vi "Item_OnPopupMenu.vi"(11 "Object":T1) -> ()   [LabVIEW 2020, in "Actor Message Maker Provider.lvlib"]
uses:
  Actor Message Maker Provider.lvlib
  <resource>/Framework/Providers/API/mxLvMenuItem.ctl
  MessageMakerProvider/Support/Localized Strings.vi
  MessageMakerProvider/Message Maker Provider.lvlib
  MessageMakerProvider/AFPP Shared/Validation Mode.ctl
  MessageMakerProvider/AFPP Shared/AFPP Shared.lvlib
  <resource>/Framework/Providers/API/ItemRef.ctl
panel:
  out "error out":errorcluster
  in  "error in":errorcluster
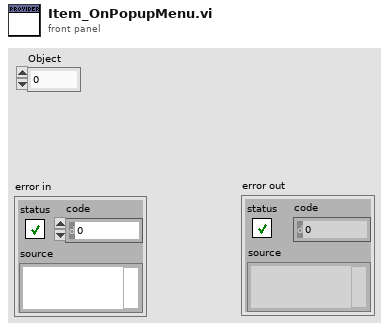
[diagram p1: front panel]
types:
  T1 = typedef "ItemRef.ctl" = u64
  T2 = typedef "AFPP Shared.lvlib/Validation Mode.ctl" = enum16{"An Actor Library", "A Target Tag"}
  T3 = typedef "mxLvMenuItem.ctl" = cluster{"Menu Name":string, "Description":string, "Icon File Name":path, "Menu Tag":string, "Enabled":bool, "Checked":bool, "Separator":bool, "Batchable":bool, "Weight":i32, "Batch Mode (Ignored if Not Batchable)":enum32{"Show If All Items Support Command", "Show If Any Items Support Command"}, "Menu Location":enum32{"<None>", "Project", "Project / Build Specifications", "Tools", "Tools / Source Control", "Tools / Real-Time Module", "Help"}, "Exclude From Getting Started Window Menu":bool}
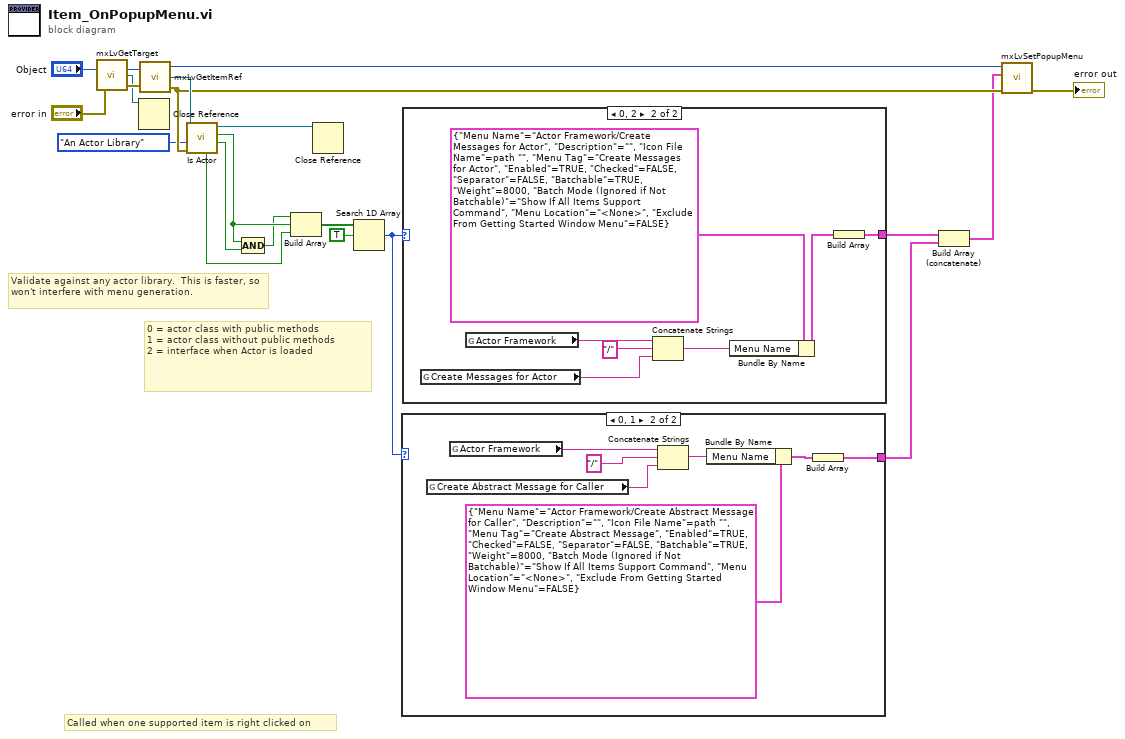
[diagram p0: block diagram]
diagram:
  # "0 = actor class with public methods\n1 = actor class without public methods\n2 = interface when Actor is loaded"
  # "Validate against any actor library.  This is faster, so won't interfere with menu generation."
  # "Called when one supported item is right clicked on"
  n1 = call <resource>:"mxLvGetTarget.vi"("Item"="Object", "error in"="error in") -> ("Item"=w10:T1, "Target"=w7:refnum<vi>, "error out"=w8:errorcluster)
  n2 = Close Reference(reference=w7) -> ()  [unwired: 1 in, 1 out]
  n3 = call <resource>:"mxLvGetItemRef.vi"("Item"=w10, "error in"=w8) -> ("Item"=w20:T1, "Item Refnum"=w18:refnum<vi>, "error out"=w17:errorcluster)
  n4 = call "Is Actor.vi"("error in (no error)"=w17, "Validation"=Validation_Mode."An Actor Library", "ProjectItem in"=w18) -> ("Has Public Methods"=w12:bool, "Is Actor"=w16:bool, "ProjectItem out"=w19:refnum<vi>, "Is Actor Interface"=w5:bool)  [unwired: 4 in, 1 out]
  n5 = Compound Arithmetic op=AND(w16, w12) -> (w15:bool)
  n6 = Build Array(w15, w16, w5) -> (w14:bool[])
  n7 = Close Reference(reference=w19) -> ()  [unwired: 1 in, 1 out]
  n8 = Search 1D Array(1D array=w14, element=TRUE) -> (index of element=w4:i32)  [unwired: 1 in]
  n9 = case shown="0, 1" w4 {
    tunnel: [_ w22] -> w2
    frame Default {
    }
    frame 0, 1 {
      n10 = global read "Localized Strings.vi" "Create Abstract Message for Caller"() -> (w26:string)
      n11 = global read "Localized Strings.vi" "Actor Framework"() -> (w25:string)
      n12 = Concatenate Strings(w25, "/", w26) -> (w27:string)
      n13 = Bundle By Name(cluster=T3 {"Menu Name"="Actor Framework/Create Abstract Message for Caller", "Description"="", "Icon File Name"=path "", "Menu Tag"="Create Abstract Message", "Enabled"=TRUE, "Checked"=FALSE, "Separator"=FALSE, "Batchable"=TRUE, "Weight"=8000, "Batch Mode (Ignored if Not Batchable)"=enum."Show If All Items Support Command", "Menu Location"=enum."<None>", "Exclude From Getting Started Window Menu"=FALSE} ("Menu Item"), "Menu Name"=w27) -> (w23:T3)
      n14 = Build Array(w23) -> (w22:T3[])
    }
  }
  n15 = case shown="0, 2" w4 {
    tunnel: [_ w33] -> w3
    frame Default {
    }
    frame 0, 2 {
      n16 = global read "Localized Strings.vi" "Create Messages for Actor"() -> (w32:string)
      n17 = global read "Localized Strings.vi" "Actor Framework"() -> (w29:string)
      n18 = Concatenate Strings(w29, "/", w32) -> (w31:string)
      n19 = Bundle By Name(cluster=T3 {"Menu Name"="Actor Framework/Create Messages for Actor", "Description"="", "Icon File Name"=path "", "Menu Tag"="Create Messages for Actor", "Enabled"=TRUE, "Checked"=FALSE, "Separator"=FALSE, "Batchable"=TRUE, "Weight"=8000, "Batch Mode (Ignored if Not Batchable)"=enum."Show If All Items Support Command", "Menu Location"=enum."<None>", "Exclude From Getting Started Window Menu"=FALSE} ("Menu Item"), "Menu Name"=w31) -> (w34:T3)
      n20 = Build Array(w34) -> (w33:T3[])
    }
  }
  n21 = Build Array (concatenate)(w3, w2) -> (w1:T3[])
  n22 = call <resource>:"mxLvSetPopupMenu.vi"("error in"=w17, "Popup Menu Items"=w1, "Item"=w20) -> ("error out"=→"error out":errorcluster)  [unwired: 7 in, 1 out]
